vi "Get UI Ref.vi"(8 "error in":errorcluster, 11 "9226 in":refnum<class "9226.lvclass">) -> (0 "error out":errorcluster, 1 "Show SubPanel?":bool, 2 "UI VI Refnum":refnum<vi>, 3 "9226 out":refnum<class "9226.lvclass">)   [LabVIEW 2017, in "Modules.lvlib" / "9226.lvclass"]
uses:
  9226.lvclass
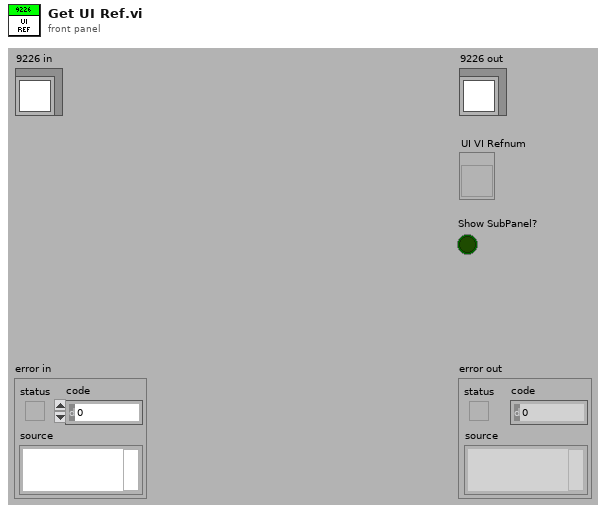
[diagram p1: front panel]
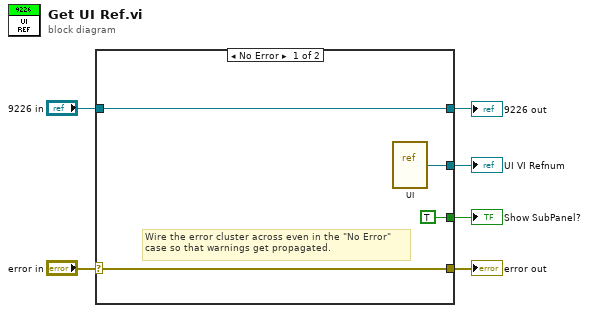
[diagram p0: block diagram]
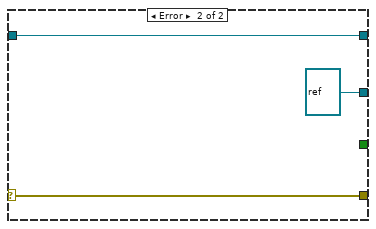
[diagram p2: hidden frame]
diagram:
  n1 = case shown="No Error" "error in" {
    selector: "error in" -> [w9 w13]
    tunnel: [w9 w13] -> w3
    tunnel: [w10 w12] -> w5
    tunnel: "9226 in" -> [w10 w12]
    tunnel: [w8 refnum<vi> refnum] -> w2
    tunnel: [TRUE _] -> w1
    frame No Error {
      # "Wire the error cluster across even in the \"No Error\"\ncase so that warnings get propagated."
      n2 = vi-ref "UI.vi"() -> (w8:refnum<vi>)
    }
    frame Error {
    }
  }
  "error out" <- w3
  "9226 out" <- w5
  "UI VI Refnum" <- w2
  "Show SubPanel?" <- w1
